vi "Queue Comms FGV.vi"(8 "Error In":errorcluster, 10 "Queue Option":T1, 11 "Queue In":refnum<queue>) -> (0 "Error Out":errorcluster, 3 "Out":refnum<queue>)   [LabVIEW 2015, in "Wash Display Console.lvlib"]
doc: "VI used to set, get or release a queue Ref."
uses:
  Wash Display Console.lvlib
  Private Controls/Queue FGV Action.ctl
  Private Controls/Module Data Cluster.ctl
  Private Controls/Module Action.ctl
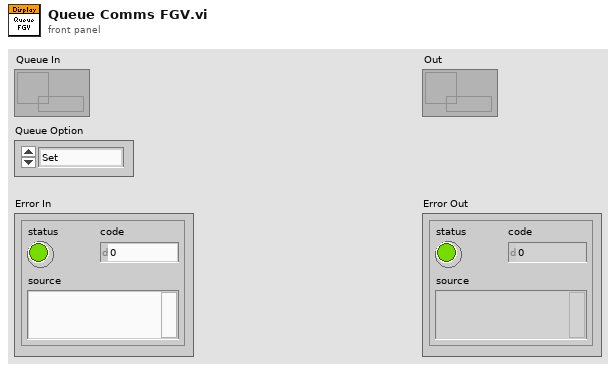
[diagram p1: front panel]
types:
  T1 = typedef "Wash Display Console.lvlib/Queue FGV Action.ctl" = enum16{"Set", "Get", "Release"}
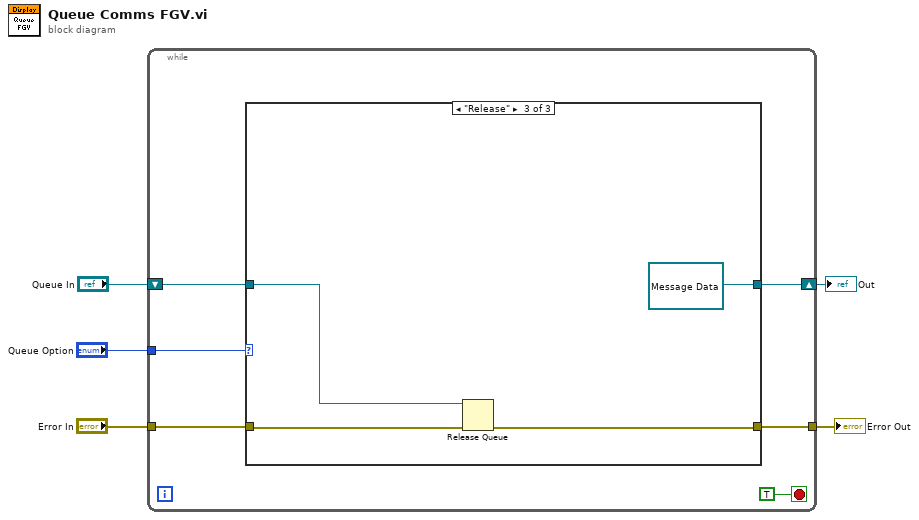
[diagram p0: block diagram]
diagram:
  n1 = while {
    tunnel: "Queue Option" -> [w10]
    tunnel: [w9] -> w4
    tunnel: "Error In" -> [w8]
    shift-right: [w6] -> w1
    shift-left: "Queue In" -> [w7]
    stop <- TRUE stop-if-true
    n2 = case shown="\"Release\"" w10 {
      tunnel: [w13 w15 w18] -> w9
      tunnel: w8 -> [w13 w15 w19]
      tunnel: w7 -> [w12 w14 w17]
      tunnel: [w12 w14 refnum<queue> refnum ("Queue In")] -> w6
      frame "Set" {
      }
      frame "Get", Default {
      }
      frame "Release" {
        n3 = Release Queue(queue=w17, error in (no error)=w19) -> (error out=w18:errorcluster)  [unwired: 1 in, 2 out]
      }
    }
  }
  "Error Out" <- w4
  "Out" <- w1
